vi "Actor Core.vi"(8 "error in":errorcluster, 11 "For Loop Dialog In":refnum<class "Subroutine Dialog.lvclass">) -> (0 "error out":errorcluster, 3 "Actor out":refnum<class "Actor.lvclass">)   [LabVIEW 2017, in "Subroutine Dialog.lvclass"]
doc: "(<B>Filename</B>: Actor Framework.lvlib:Actor.lvclass:Actor Core.vi)\n\nReceives messages to the actor, reacts to them, and initiates any error handling that may shut the actor down.\n\nDescendant classes may override this VI to append parallel tasks for the actor to complete while it handles messages. Overrides use the Call Parent Method node.\n\n<License>\nCopyright © 2017 Composed Systems, LLC | All rights reserved\nwww.composed.io\n\nAuthor: Ethan Stern <ethan.stern@composed.io>\n\nThis software is provided \"AS IS\" WITHOUT WARRANTIES, either express or implied, AND IS FOR EDUCATIONAL PURPOSES ONLY.\n</License>"
uses:
  Subroutine Dialog.lvclass
  ITest Executive Builder Dialog/ITest Executive Builder Dialog.lvclass
  <vilib>/gpm_packages/@cs/mva-viewable/Source/ActorEvents/IEventAggregator/IEventAggregator.lvclass
  <vilib>/event_ctls.llb/lveventtype.ctl
  <vilib>/gpm_packages/@cs/mva-viewable/Source/IViewable/ProtectedSubpanel/ProtectedSubpanel.lvclass
  C:/Users/jonmc/Documents/Git/Test Executive Builder/Source/Test Executive Builder Dialogs/ITest Executive Builder Dialog/ITest Executive Builder Dialog.lvclass
  C:/Users/jonmc/Documents/Git/Test Executive Builder/gpm_packages/@cs/mva-viewable/Source/ActorEvents/IEventAggregator/IEventAggregator.lvclass
  <vilib>/ActorFramework/Actor/Actor.lvclass
panel:
  in  "Attribute Notes":string
  in  "Attribute Name":u16(ring)
  in  "Restore Point":bool
  in  "Cancel":bool
  in  "OK":bool
  in  "Subroutine Name":string
  in  "Tab Control":enum32{"Value", "Pointer"}(tab)
  in  "Pointer":u16(ring)
  # "Edit Subroutine"
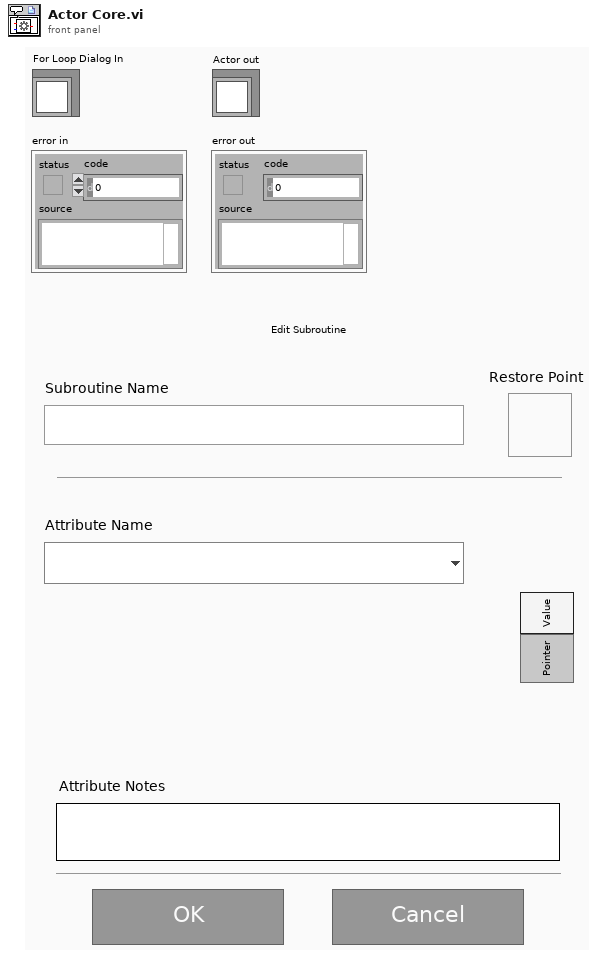
[diagram p1: front panel]
types:
  T1 = typedef "lveventtype.ctl" = enum32{"Null", "Timeout", "Annotation Menu Selection", "Annotation Menu Selection?", "App Instance Close", "App Instance Close?", "Autoscale Range Change", "Bookmark Info Change", "Cell Edit", "Cell Edit?", "Cursor Grab", "Cursor Grab?", "Cursor Menu Selection", "Cursor Menu Selection?", "Cursor Move", "Cursor Release", "Data Change", "Direction Change", "Display State Change", "Drag Ended", "Drag Enter", "Drag Leave", "Drag Over", "Drag Source Update", "Drag Starting", "Drag Starting?", "Drop", "Exec State Change", "Key Down", "Key Down?", "Key Repeat", "Key Repeat?", "Key Up", "Listbox Double Click", "Menu Activation?", "Menu Selection (App)", "Menu Selection? (App)", "Menu Selection (User)", "Mouse Down", "Mouse Down?", "Mouse Enter", "Mouse Leave", "Mouse Move", "Mouse Up", "Mouse Wheel", "NI Security User Change (App)", "Pane Size", "Panel Close", "Panel Close?", "Panel Resize", "Plot Attribute Change", "Scale Range Change", "Shortcut Menu Activation?", "Shortcut Menu Selection (App)", "Shortcut Menu Selection? (App)", "Shortcut Menu Selection (User)", "Tree Double Click", "Tree Drag", "Tree Drag?", "Tree Drop", "Tree Drop?", "Tree Item Close", "Tree Item Close?", "Tree Item Open", "Tree Item Open?", "User Event", "Value Change"}
  T2 = typedef "IViewable.lvlib/ProtectedSubpanel.lvclass/Protected Subpanel Reference.ctl" = refnum<data-value>
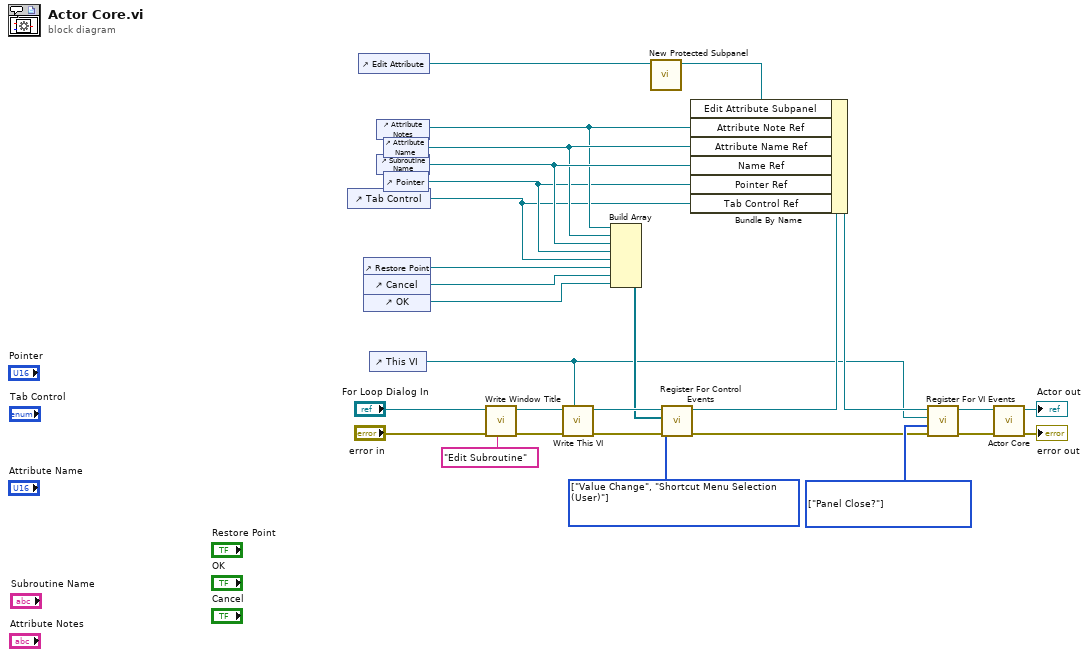
[diagram p0: block diagram]
diagram:
  w15 = T1[] [enum."Panel Close?"] items=["Null", "Timeout", "Annotation Menu Selection", "Annotation Menu Selection?", "App Instance Close", "App Instance Close?", "Autoscale Range Change", "Bookmark Info Change", "Cell Edit", "Cell Edit?", "Cursor Grab", "Cursor Grab?", "Cursor Menu Selection", "Cursor Menu Selection?", "Cursor Move", "Cursor Release", "Data Change", "Direction Change", "Display State Change", "Drag Ended", "Drag Enter", "Drag Leave", "Drag Over", "Drag Source Update", "Drag Starting", "Drag Starting?", "Drop", "Exec State Change", "Key Down", "Key Down?", "Key Repeat", "Key Repeat?", "Key Up", "Listbox Double Click", "Menu Activation?", "Menu Selection (App)", "Menu Selection? (App)", "Menu Selection (User)", "Mouse Down", "Mouse Down?", "Mouse Enter", "Mouse Leave", "Mouse Move", "Mouse Up", "Mouse Wheel", "NI Security User Change (App)", "Pane Size", "Panel Close", "Panel Close?", "Panel Resize", "Plot Attribute Change", "Scale Range Change", "Shortcut Menu Activation?", "Shortcut Menu Selection (App)", "Shortcut Menu Selection? (App)", "Shortcut Menu Selection (User)", "Tree Double Click", "Tree Drag", "Tree Drag?", "Tree Drop", "Tree Drop?", "Tree Item Close", "Tree Item Close?", "Tree Item Open", "Tree Item Open?", "User Event", "Value Change"] ("Registration Types")
  w21 = T1[] [enum."Value Change", enum."Shortcut Menu Selection (User)"] items=["Null", "Timeout", "Annotation Menu Selection", "Annotation Menu Selection?", "App Instance Close", "App Instance Close?", "Autoscale Range Change", "Bookmark Info Change", "Cell Edit", "Cell Edit?", "Cursor Grab", "Cursor Grab?", "Cursor Menu Selection", "Cursor Menu Selection?", "Cursor Move", "Cursor Release", "Data Change", "Direction Change", "Display State Change", "Drag Ended", "Drag Enter", "Drag Leave", "Drag Over", "Drag Source Update", "Drag Starting", "Drag Starting?", "Drop", "Exec State Change", "Key Down", "Key Down?", "Key Repeat", "Key Repeat?", "Key Up", "Listbox Double Click", "Menu Activation?", "Menu Selection (App)", "Menu Selection? (App)", "Menu Selection (User)", "Mouse Down", "Mouse Down?", "Mouse Enter", "Mouse Leave", "Mouse Move", "Mouse Up", "Mouse Wheel", "NI Security User Change (App)", "Pane Size", "Panel Close", "Panel Close?", "Panel Resize", "Plot Attribute Change", "Scale Range Change", "Shortcut Menu Activation?", "Shortcut Menu Selection (App)", "Shortcut Menu Selection? (App)", "Shortcut Menu Selection (User)", "Tree Double Click", "Tree Drag", "Tree Drag?", "Tree Drop", "Tree Drop?", "Tree Item Close", "Tree Item Close?", "Tree Item Open", "Tree Item Open?", "User Event", "Value Change"] ("Registration Types")
  n1 = control-ref of="Tab Control"() -> (w2:refnum<vi>)
  n2 = control-ref of="Edit Attribute"() -> (w1:refnum<vi>)
  n3 = control-ref of="Restore Point"() -> (w5:refnum<vi>)
  n4 = control-ref of="Cancel"() -> (w20:refnum<vi>)
  n5 = control-ref of="OK"() -> (w19:refnum<vi>)
  n6 = control-ref of="This VI"() -> (w10:refnum<vi>)
  n7 = control-ref of="Attribute Notes"() -> (w4:refnum<vi>)
  n8 = control-ref of="Subroutine Name"() -> (w18:refnum<vi>)
  n9 = control-ref of="Attribute Name"() -> (w17:refnum<vi>)
  n10 = control-ref of="Pointer"() -> (w3:refnum<vi>)
  n11 = call "Write Window Title.vi"("Window Title"="Edit Subroutine", "ITest Executive Builder Dialog in"="For Loop Dialog In") -> ("ITest Executive Builder Dialog out"=w8:refnum<class "Subroutine Dialog.lvclass">)  [unwired: 9 in]
  n12 = call "Write This VI.vi"("This VI"=w10, "ITest Executive Builder Dialog in"=w8) -> ("ITest Executive Builder Dialog out"=w23:refnum<class "Subroutine Dialog.lvclass">)  [unwired: 9 in]
  n13 = Build Array(w4, w17, w18, w3, w2, w5, w20, w19) -> (w16:refnum<vi>[])
  n14 = call <vilib>:"New Protected Subpanel.vi"("SubPnl Refnum"=w1) -> ("Protected Subpanel"=w6:T2)  [unwired: 9 in, 1 out]
  n15 = call <vilib>:"Register For Control Events.vi"("error in (no error)"="error in", "Registration Types"=w21, "Control Refnums"=w16, "IEventAggregator In"=w23) -> ("error out"=w14:errorcluster, "IEventAggregator Out"=w22:refnum<class "Subroutine Dialog.lvclass">)  [unwired: 6 in]
  n16 = Bundle By Name(cluster=w22, "Edit Attribute Subpanel"=w6, "Attribute Note Ref"=w4, "Attribute Name Ref"=w17, "Name Ref"=w18, "Pointer Ref"=w3, "Tab Control Ref"=w2) -> (w12:refnum<class "Subroutine Dialog.lvclass">)
  n17 = call <vilib>:"Register For VI Events.vi"("error in (no error)"=w14, "Registration Types"=w15, "VI Refnum"=w10, "IEventAggregator In"=w12) -> ("error out"=w13:errorcluster, "IEventAggregator Out"=w11:refnum<class "Subroutine Dialog.lvclass">)  [unwired: 6 in]
  n18 = call-parent "Actor Core.vi"("error in"=w13, "ITest Executive Builder Dialog In"=w11) -> ("error out"=→"error out":errorcluster, "Actor out"=→"Actor out":refnum<class "Actor.lvclass">)  [unwired: 8 in]
